vi "Make cell folder.vi"(1 "Error bundle in.":errorcluster, 2 "Cell folder number.":dbl format="%.2f", 3 "Ear folder path name.":path, 4 "Ear folder path name (string).":string) -> (0 "Error bundle out.":errorcluster)   [LabVIEW 2010]
panel:
  # "Inputs:"
  # "Outputs:"
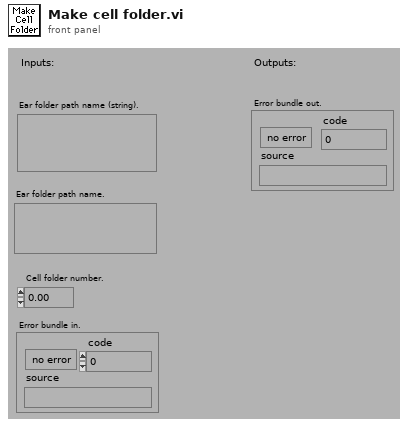
[diagram p1: front panel]
types:
  T1 = enum16{"open", "replace", "create", "open or create", "replace or create", "replace or create with confirmation"}
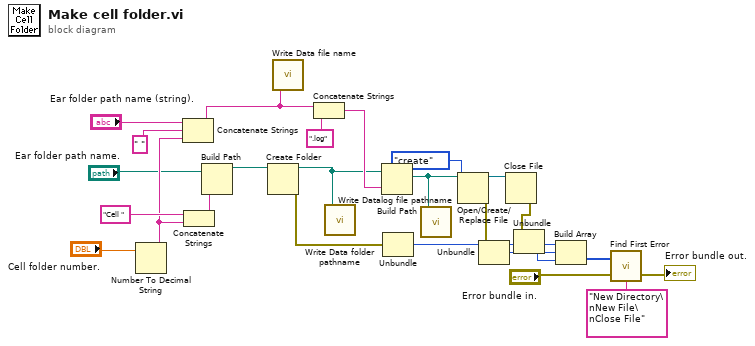
[diagram p0: block diagram]
diagram:
  n1 = Number To Decimal String(number="Cell folder number.") -> (decimal integer string=w21:string)  [unwired: 1 out]
  n2 = Concatenate Strings("Ear folder path name (string).", " ", w21) -> (w15:string)
  n3 = Concatenate Strings("Cell ", w21) -> (w24:string)
  n4 = Build Path(base path="Ear folder path name.", name or relative path=w24) -> (appended path=w25:path)
  n5 = Create Folder(path (use dialog)=w25) -> (created path=w16:path, error out=w12:errorcluster)  [unwired: 1 in, 2 out]
  n6 = call "Write Data file name.vi"("Data file name."=w15) -> ()  [unwired: 1 out]
  n7 = Concatenate Strings(w15, ".log") -> (w18:string)
  n8 = call "Write Data folder pathname.vi"("Data folder pathname."=w16) -> ()  [unwired: 1 out]
  n9 = Build Path(base path=w16, name or relative path=w18) -> (appended path=w19:path)
  n10 = Unbundle(w12) -> ("code"=w2:i32)  [unwired: 2 out]
  n11 = call "Write Datalog file pathname.vi"("Datalog file pathname."=w19) -> ()  [unwired: 1 out]
  n12 = Open/Create/Replace File(file path (use dialog)=w19, operation (0:open)=T1."create") -> (refnum out=w17:refnum<file>, error out=w11:errorcluster)  [unwired: 1 in, 4 out]
  n13 = Unbundle(w11) -> ("code"=w3:i32)  [unwired: 2 out]
  n14 = Close File(refnum=w17) -> (error out=w10:errorcluster)  [unwired: 1 in, 1 out]
  n15 = Unbundle(w10) -> ("code"=w4:i32)  [unwired: 2 out]
  n16 = Build Array(w2, w3, w4) -> (w9:i32[])
  n17 = call <vilib>:"Find First Error.vi"("error in (no error)"="Error bundle in.", "source messages"="New Directory\nNew File\nClose File", "error codes"=w9) -> ("error out"=→"Error bundle out.":errorcluster)  [unwired: 2 out]
